vi "Safety_Check.vi"(1 "Adam Loop Count":i32, 2 "Ch Names":string[](array[string]), 3 "Values":dbl[](array[numeric]) format="%.2f") -> (0 "Scan comment":string)   [LabVIEW 2012]
uses:
  ADAM Client/Sub VIs/ADAM Controls/Update_scan_value.ctl
  Anemometry/Anemometry Sub Vis/Globals/Gas_management_global.vi
  ADAM_Global.vi
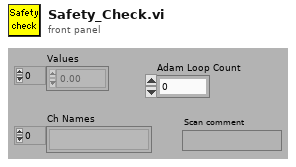
[diagram p1: front panel]
types:
  T1 = cluster{"Channel name":string, "Set value of A to":dbl, "Set value of B to":dbl, "Set value of C to":dbl, "Set value of D to":dbl}
  T2 = typedef "Update_scan_value.ctl" = cluster{"Channel Name":string, "New Value":dbl}
  T3 = enum16{"Append to Global", "Read Global then Clear"}
  T4 = enum16{"On", "Off", "Always On", "Always Off", "Delete"}
  T5 = typedef "LVDateTimeRec.ctl" = cluster{"fractional second":dbl, "second":i32, "minute":i32, "hour":i32, "day of month":i32, "month":i32, "year":i32, "day of week":i32, "day of year":i32, "DST":i32}
  T6 = cluster{"Channel name":string, "Set value of A to":dbl, "Set value of B to":dbl, "Set value of C to":dbl, "Set value of D to":dbl}[]
  T7 = typedef "Ch_description_ADAM.ctl" = cluster{"Ch Name":string, "Type":T8, "Function":T9, "Ch State":T10, "Calibration type":T11, "A":dbl, "B":dbl, "C":dbl, "D":dbl, "Comments":string, "Address":T12, "String":string, "Duty":u16}
  T8 = typedef "Module_type_ADAM.ctl" = string
  T9 = typedef "Function_ADAM.ctl" = enum16{"Analogue Input", "Digital Input", "Event counter", "Event rate", "Analogue Output", "Digital Output", "Relay Output"}
  T10 = typedef "Channel_State.ctl" = enum16{"On", "Off", "Always On", "Always Off"}
  T11 = typedef "Calib_type_ADAM.ctl" = enum16{"Raw", "Bx + A", "Cx^2 + Bx + A", "Dx^3 + Cx^2 + Bx + A", "In Band", "Hi-Tec Q", "Hi-Tec M_dot", "Text"}
  T12 = typedef "Address.ctl" = cluster{"Main":i32, "Ch.":i32, "Sub":i32, "Port Name":string}
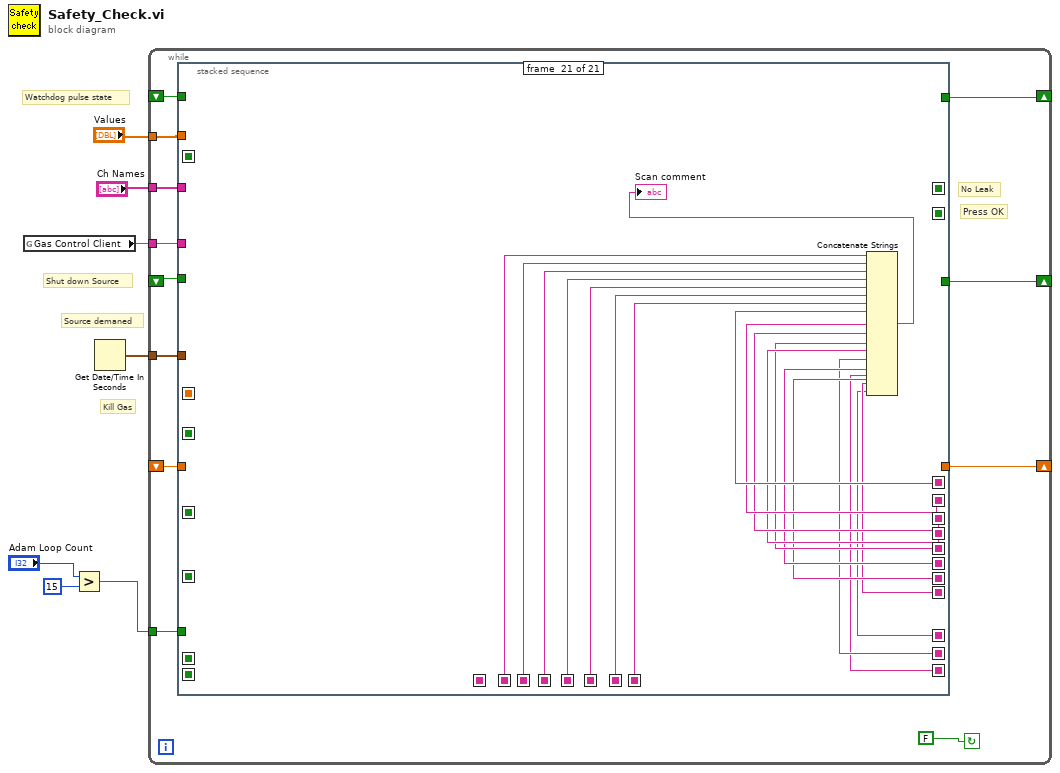
[diagram p0: block diagram]
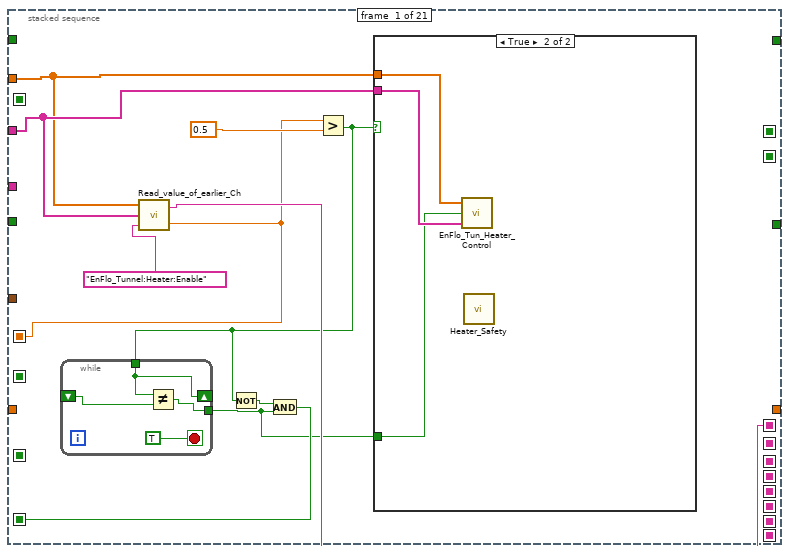
[diagram p2: hidden frame]
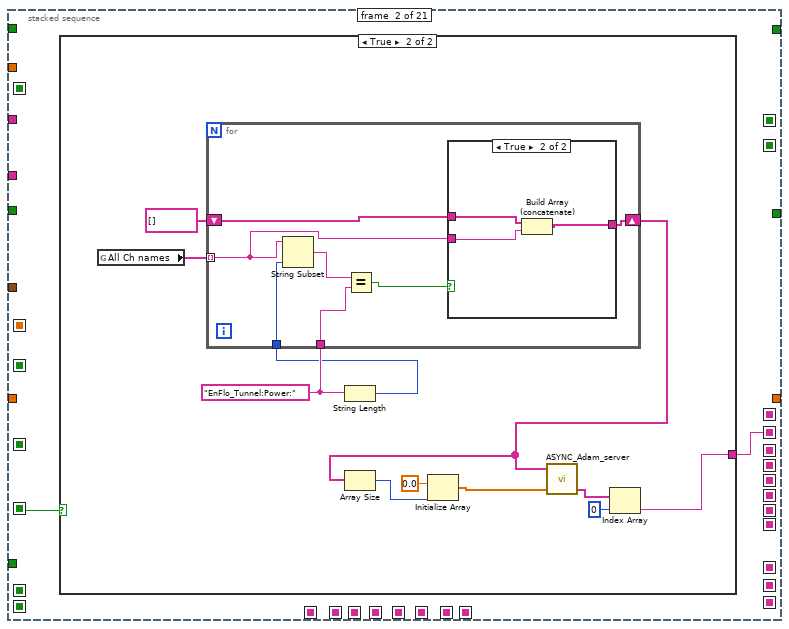
[diagram p4: hidden frame]
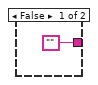
[diagram p5: hidden frame]
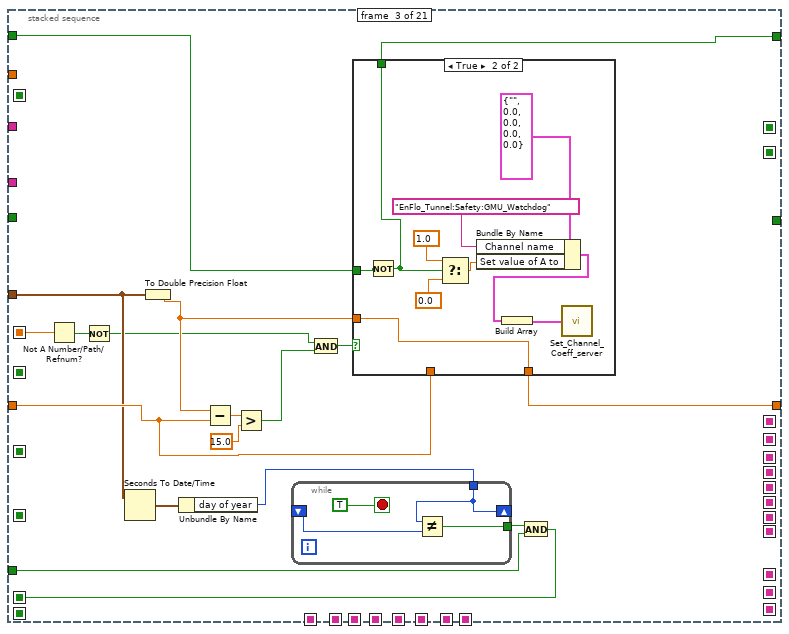
[diagram p7: hidden frame]
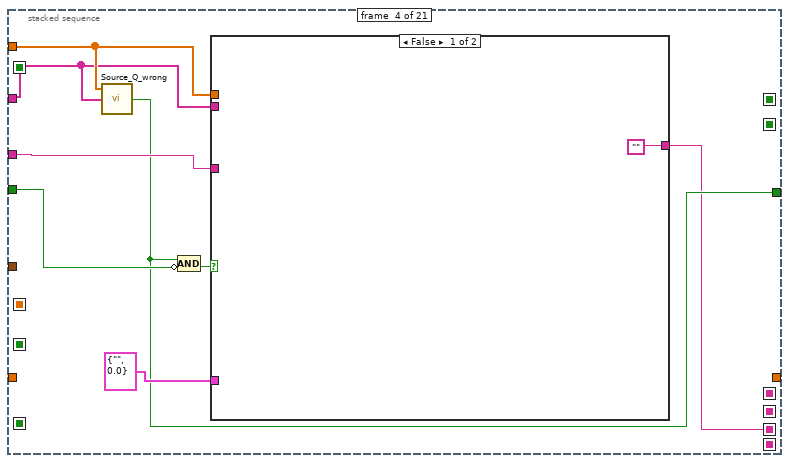
[diagram p9: hidden frame]
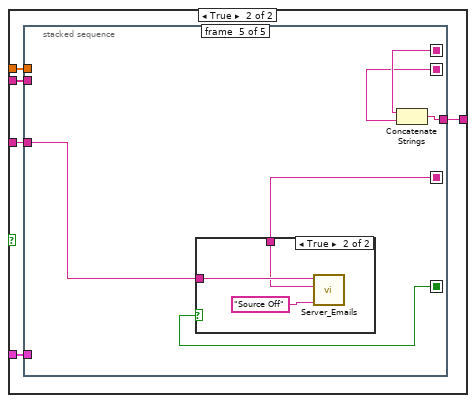
[diagram p10: hidden frame]
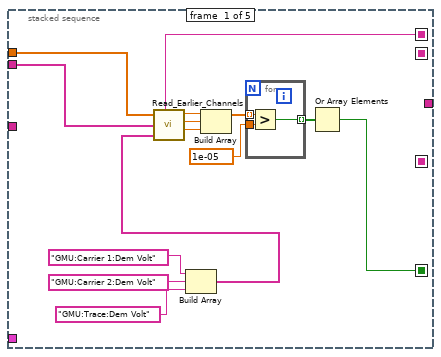
[diagram p11: hidden frame]
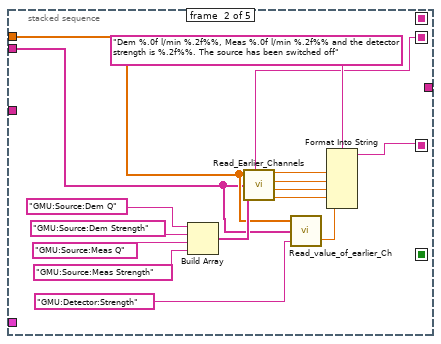
[diagram p12: hidden frame]
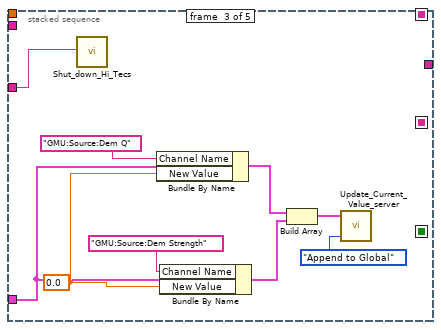
[diagram p13: hidden frame]
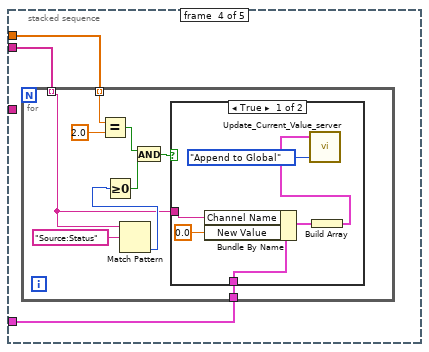
[diagram p14: hidden frame]
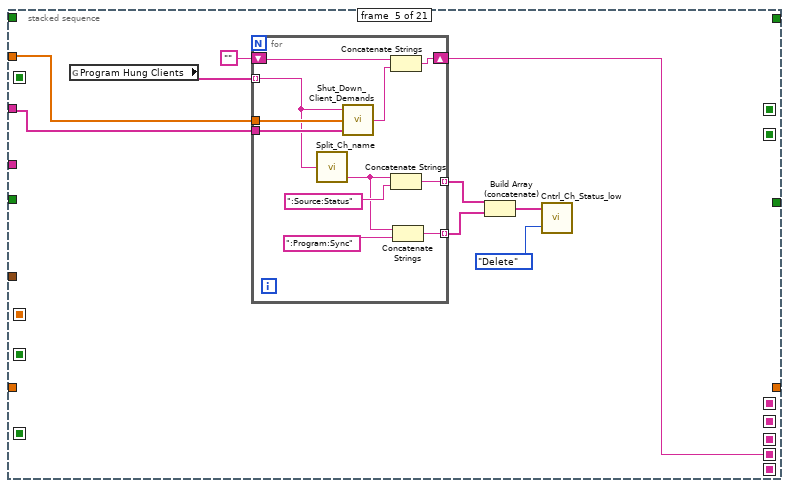
[diagram p17: hidden frame]
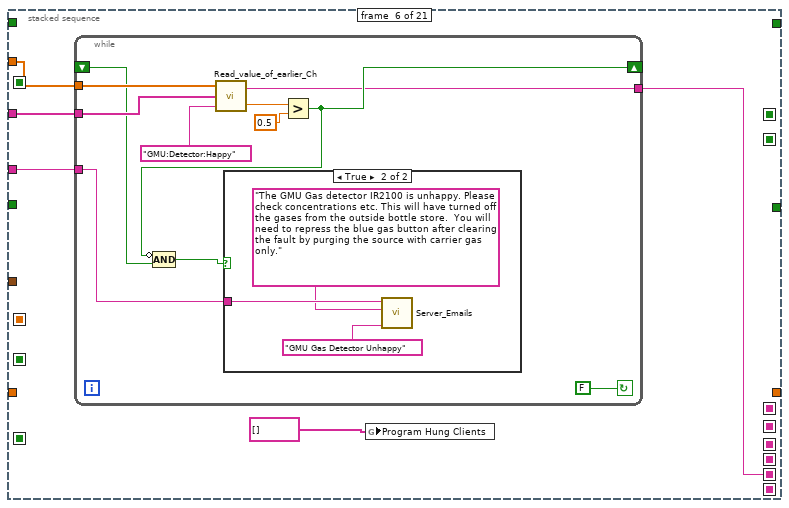
[diagram p18: hidden frame]
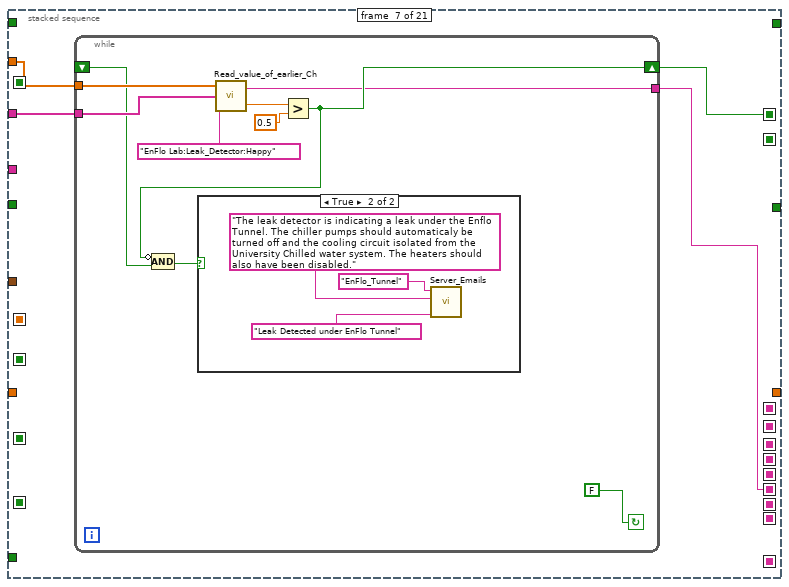
[diagram p20: hidden frame]
diagram:
  # "Shut down Source"
  # "Source demaned"
  # "Watchdog pulse state"
  # "Kill Gas"
  n1 = global read "Gas_management_global.vi" "Gas Control Client"() -> (w5:string)
  n2 = Greater?(x="Adam Loop Count", y=15) -> (0:w2:bool)
  n3 = Get Date/Time In Seconds() -> (seconds since 1Jan1904=w1:timestamp)
  n4 = while {
    shift-left: _ -> [w14]
    shift-right: [w13] -> _
    shift-left: _ -> [w16]
    shift-right: [w15] -> _
    tunnel: w5 -> [w18]
    tunnel: "Ch Names" -> [w19]
    tunnel: "Values" -> [w17]
    shift-right: [w11] -> _
    shift-left: _ -> [w10]
    tunnel: w2 -> [w9]
    tunnel: w1 -> [w8]
    stop <- FALSE continue-if-true
    # "Press OK"
    # "No Leak"
    n5 = stacked-sequence {
      seq-local: [_ _ _ _ _ _ w219 _ _ _ _ _ _ _ _ _ _ _ _ _ _] -> [_ _ _ _ _ _ _ _ _ _ _ _ _ w448 _ _ _ _ _ _ _]
      seq-local: [w22 _ _ _ _ _ _ _ _ _ _ _ _ _ _ _ _ _ _ _ _] -> [_ w38 _ _ _ _ _ _ _ _ _ _ _ _ _ _ _ _ _ _ _]
      seq-local: [_ _ w68 _ _ _ _ _ _ _ _ _ _ _ _ _ _ _ _ _ _] -> [_ _ _ _ _ _ _ _ _ _ _ _ _ _ _ _ _ _ _ _ _]
      seq-local: [_ _ _ _ _ _ _ _ _ _ _ _ _ _ _ w509 _ _ _ _ _] -> [_ _ _ _ _ _ _ _ _ _ _ _ _ _ _ _ w525 _ _ _ _]
      seq-local: [_ _ _ _ _ _ _ _ _ _ _ _ _ _ _ _ w517 _ _ _ _] -> [_ _ _ _ _ _ _ _ _ _ _ _ _ _ _ _ _ _ _ w649 _]
      seq-local: [w25 _ _ _ _ _ _ _ _ _ _ _ _ _ _ _ _ _ _ _ _] -> [_ _ _ _ _ _ _ _ _ _ _ _ _ _ _ _ _ _ _ _ w686]
      seq-local: [_ w37 _ _ _ _ _ _ _ _ _ _ _ _ _ _ _ _ _ _ _] -> [_ _ _ _ _ _ _ _ _ _ _ _ _ _ _ _ _ _ _ _ w685]
      seq-local: [_ _ _ w96 _ _ _ _ _ _ _ _ _ _ _ _ _ _ _ _ _] -> [_ _ _ _ _ _ _ _ _ _ _ _ _ _ _ _ _ _ _ _ w684]
      seq-local: [_ _ _ _ w179 _ _ _ _ _ _ _ _ _ _ _ _ _ _ _ _] -> [_ _ _ _ _ _ _ _ _ _ _ _ _ _ _ _ _ _ _ _ w683]
      seq-local: [_ _ _ _ _ w199 _ _ _ _ _ _ _ _ _ _ _ _ _ _ _] -> [_ _ _ _ _ _ _ _ _ _ _ _ _ _ _ _ _ _ _ _ w682]
      seq-local: [_ _ _ _ _ _ w218 _ _ _ _ _ _ _ _ _ _ _ _ _ _] -> [_ _ _ _ _ _ _ _ _ _ _ _ _ _ _ _ _ _ _ _ w681]
      seq-local: [_ _ _ _ _ _ _ _ _ w326 _ _ _ _ _ _ _ _ _ _ _] -> [_ _ _ _ _ _ _ _ _ _ _ _ _ _ _ _ _ _ _ _ w680]
      seq-local: [_ _ _ _ _ _ _ _ _ _ w358 _ _ _ _ _ _ _ _ _ _] -> [_ _ _ _ _ _ _ _ _ _ _ _ _ _ _ _ _ _ _ _ w671]
      seq-local: [_ _ _ _ _ _ _ _ _ _ _ _ w425 _ _ _ _ _ _ _ _] -> [_ _ _ _ _ _ _ _ _ _ _ _ _ _ _ _ _ _ _ _ w670]
      seq-local: [_ _ _ _ _ _ _ _ _ _ _ _ _ w449 _ _ _ _ _ _ _] -> [_ _ _ _ _ _ _ _ _ _ _ _ _ _ _ _ _ _ _ _ w673]
      seq-local: [_ _ _ _ _ _ _ _ _ _ _ _ _ _ w476 _ _ _ _ _ _] -> [_ _ _ _ _ _ _ _ _ _ _ _ _ _ _ _ _ _ _ _ w674]
      seq-local: [_ _ _ _ _ _ _ _ _ _ _ _ _ _ _ w500 _ _ _ _ _] -> [_ _ _ _ _ _ _ _ _ _ _ _ _ _ _ _ _ _ _ _ w675]
      seq-local: [_ _ _ _ _ _ _ _ _ _ _ _ _ _ _ _ w514 _ _ _ _] -> [_ _ _ _ _ _ _ _ _ _ _ _ _ _ _ _ _ _ _ _ w676]
      seq-local: [_ _ _ _ _ _ _ _ _ _ _ _ _ _ _ _ _ w582 _ _ _] -> [_ _ _ _ _ _ _ _ _ _ _ _ _ _ _ _ _ _ _ _ w677]
      seq-local: [_ _ _ _ _ _ _ _ _ _ _ _ _ _ _ _ _ _ w611 _ _] -> [_ _ _ _ _ _ _ _ _ _ _ _ _ _ _ _ _ _ _ _ w678]
      seq-local: [_ _ _ _ _ _ _ _ _ _ _ _ _ _ _ _ _ _ _ w647 _] -> [_ _ _ _ _ _ _ _ _ _ _ _ _ _ _ _ _ _ _ _ w679]
      seq-local: [w24 _ _ _ _ _ _ _ _ _ _ _ _ _ _ _ _ _ _ _ _] -> [_ _ w66 _ _ _ _ _ _ _ _ _ _ _ _ _ _ _ _ _ _]
      seq-local: [_ _ _ _ _ _ _ _ _ _ _ _ _ _ _ w499 _ _ _ _ _] -> [_ _ _ _ _ _ _ _ _ _ _ _ _ _ _ _ w513 _ _ _ _]
      seq-local: [_ _ _ _ _ _ _ w237 _ _ _ _ _ _ _ _ _ _ _ _ _] -> [_ _ _ _ _ _ _ _ _ _ _ _ _ w447 _ _ _ _ _ _ _]
      seq-local: [_ _ _ _ _ _ _ w236 _ _ _ _ _ _ _ _ _ _ _ _ _] -> [_ _ _ _ _ _ _ _ _ _ _ _ _ _ _ _ _ _ _ _ w669]
      seq-local: [_ _ _ _ _ _ _ w235 _ _ _ _ _ _ _ _ _ _ _ _ _] -> [_ _ _ _ _ _ _ _ w267 _ _ _ _ _ _ _ _ _ _ _ _]
      seq-local: [_ _ _ _ _ _ _ _ w264 _ _ _ _ _ _ _ _ _ _ _ _] -> [_ _ _ _ _ _ _ _ _ _ _ _ _ _ _ _ _ _ _ _ _]
      seq-local: [_ _ _ _ _ _ _ _ _ _ _ w379 _ _ _ _ _ _ _ _ _] -> [_ _ _ _ _ _ _ _ _ _ _ _ _ _ _ _ _ _ _ _ w668]
      tunnel: w19 -> [w27 _ _ w98 w186 w201 w220 w238 w265 w327 w359 w380 w427 w450 w482 w505 w526 w587 w614 _ _]
      tunnel: w18 -> [_ _ _ w103 _ w200 _ _ _ _ _ _ _ _ _ _ _ _ _ _ _]
      tunnel: w17 -> [w26 _ _ w99 w182 w202 w221 w239 w266 w328 w360 w381 w428 w451 w483 w506 w527 w588 w615 _ _]
      tunnel: w16 -> [_ _ w79 _ _ _ _ _ _ _ _ _ _ _ _ _ _ _ _ _ _]
      tunnel: [_ _ w78 _ _ _ _ _ _ _ _ _ _ _ _ _ _ _ _ _ _] -> w15
      tunnel: w14 -> [_ _ _ w102 _ _ _ _ _ _ _ _ _ _ _ _ _ _ _ _ _]
      tunnel: [_ _ _ w97 _ _ _ _ _ _ _ _ _ _ _ _ _ _ _ _ _] -> w13
      tunnel: [_ _ w77 _ _ _ _ _ _ _ _ _ _ _ _ _ _ _ _ _ _] -> w11
      tunnel: w10 -> [_ _ w73 _ _ _ _ _ _ _ _ _ _ _ _ _ _ _ _ _ _]
      tunnel: w9 -> [_ _ w69 _ _ _ _ _ _ _ _ _ w426 _ _ _ w518 w583 _ w648 _]
      tunnel: w8 -> [_ _ w67 _ _ _ _ _ _ _ _ w378 _ _ _ _ _ _ _ _ _]
      frame #0 {
        n6 = call "Read_value_of_earlier_Ch.vi"("Desired Ch to Read"="EnFlo_Tunnel:Heater:Enable", "Ch names"=w27, "Present scan array"=w26) -> ("Value"=w24:dbl, "Scan comment"=w25:string)  [unwired: 1 in]
        n7 = Greater?(x=w24, y=0.5) -> (0:w23:bool)
        n8 = while {
          shift-right: [w33] -> _
          shift-left: _ -> [w32]
          tunnel: w23 -> [w33]
          tunnel: [w30] -> w20
          stop <- TRUE stop-if-true
          n9 = Not Equal?(x=w33, y=w32) -> (x != y?=w30:bool)
        }
        n10 = Not(x=w23) -> (.not. x?=w21:bool)
        n11 = And(x=w21, y=w20) -> (x .and. y?=w22:bool)
        n12 = case shown="True" w23 {
          tunnel: w26 -> [_ w36]
          tunnel: w27 -> [_ w35]
          tunnel: w20 -> [_ w34]
          frame False {
          }
          frame True {
            n13 = call "EnFlo_Tun_Heater_Control.vi"("Ch Names"=w35, "Heaters Just Enabled"=w34, "Values"=w36) -> ()  [unwired: 1 in]
            n14 = call "Heater_Safety.vi"() -> ()  [unwired: 3 in, 5 out]
          }
        }
      }
      frame #1 {
        n15 = case shown="True" w38 {
          tunnel: ["" w41] -> w37
          frame False {
          }
          frame True {
            w50 = "EnFlo_Tunnel:Power:"
            n16 = global read "ADAM_Global.vi" "All Ch names"() -> (w40:string[])
            n17 = String Length(string=w50) -> (length=w49:i32)
            n18 = for {
              shift-right: [w52] -> w45
              shift-left: string[] [] -> [w53]
              tunnel: w40 -> [w56] mode=indexing
              tunnel: w49 -> [w57]
              tunnel: w50 -> [w54]
              n19 = String Subset(string=w56, length (rest)=w57) -> (substring=w55:string)  [unwired: 1 out]
              n20 = Equal?(x=w55, y=w54) -> (x = y?=w51:bool)
              n21 = case shown="True" w51 {
                tunnel: w56 -> [_ w61]
                tunnel: w53 -> [w58 w59]
                tunnel: [w58 w60] -> w52
                frame False {
                }
                frame True {
                  n22 = Build Array (concatenate)(w59, w61) -> (w60:string[])
                }
              }
            }
            n23 = Array Size(array=w45) -> (size(s)=w46:i32)
            n24 = Initialize Array(0.0 ("element"), w46) -> (w44:dbl[])
            n25 = call "ASYNC_Adam_server.vi"("Values"=w44, "Channel Names"=w45) -> ("Scan Comments"=w43:string[])  [unwired: 1 in, 2 out]
            n26 = Index Array(array=w43, index=0) -> (element=w41:string)
          }
        }
      }
      frame #2 {
        n27 = Not A Number/Path/Refnum?(number/path/refnum=w66) -> (NaN/Path/Refnum?=w65:bool)
        n28 = Not(x=w65) -> (.not. x?=w63:bool)
        n29 = Seconds To Date/Time(time stamp (now)=w67) -> (date time rec=w72:T5)  [unwired: 1 in]
        n30 = To Double Precision Float(number=w67) -> (double precision float=w76:dbl)
        n31 = Unbundle By Name(w72) -> ("day of year"=w71:i32)
        n32 = Subtract(x=w76, y=w73) -> (x-y=w75:dbl)
        n33 = Greater?(x=w75, y=15.0) -> (0:w64:bool)
        n34 = while {
          shift-right: [w83] -> _
          shift-left: _ -> [w82]
          tunnel: w71 -> [w83]
          tunnel: [w81] -> w70
          stop <- TRUE stop-if-true
          n35 = Not Equal?(x=w83, y=w82) -> (x != y?=w81:bool)
        }
        n36 = And(x=w63, y=w64) -> (x .and. y?=w62:bool)
        n37 = case shown="True" w62 {
          tunnel: w79 -> [w84 w88]
          tunnel: [w84 w87] -> w78
          tunnel: [w85 w86] -> w77
          tunnel: w76 -> [_ w86]
          tunnel: w73 -> [w85 _]
          frame False {
          }
          frame True {
            n38 = Not(x=w88) -> (.not. x?=w87:bool)
            n39 = Select(t=1.0 ("Suction"), s=w87, f=0.0 ("Suction")) -> (s? t:f=w91:dbl)
            n40 = Bundle By Name(cluster=T1 {"Channel name"="", "Set value of A to"=0.0, "Set value of B to"=0.0, "Set value of C to"=0.0, "Set value of D to"=0.0}, "Channel name"="EnFlo_Tunnel:Safety:GMU_Watchdog" ("Desired Ch to Read"), "Set value of A to"=w91) -> (w95:T1)
            n41 = Build Array(w95) -> (w90:T6)
            n42 = call "Set_Channel_Coeff_server.vi"("Set Array"=w90) -> ()
          }
        }
        n43 = And(x=w70, y=w69) -> (x .and. y?=w68:bool)
      }
      frame #3 {
        n44 = call "Source_Q_wrong.vi"("Ch Names"=w98, "Values"=w99) -> ("Gas Error?"=w97:bool)  [unwired: 1 out]
        n45 = Compound Arithmetic op=AND(w97, invert w102) -> (w101:bool)
        n46 = case shown="False" w101 {
          tunnel: w103 -> [_ w109]
          tunnel: w99 -> [_ w108]
          tunnel: w98 -> [_ w107]
          tunnel: T2 {"Channel Name"="", "New Value"=0.0} ("Update Scan Value Cluster") -> [_ w106]
          tunnel: ["" w105] -> w96
          frame False {
          }
          frame True {
            n47 = stacked-sequence {
              seq-local: [_ w141 _ _ _] -> [_ _ _ _ w174]
              seq-local: [w111 _ _ _ _] -> [_ _ _ _ w173]
              seq-local: [w110 _ _ _ _] -> [_ _ _ _ w172]
              seq-local: [_ w127 _ _ _] -> [_ _ _ _ w171]
              tunnel: w109 -> [_ _ w144 _ w175]
              tunnel: w108 -> [w121 w131 _ w153 _]
              tunnel: w107 -> [w122 w130 _ w154 _]
              tunnel: w106 -> [_ _ w143 w152 _]
              tunnel: [_ _ _ _ w170] -> w105
              frame #0 {
                n48 = Build Array("GMU:Carrier 1:Dem Volt", "GMU:Carrier 2:Dem Volt", "GMU:Trace:Dem Volt") -> (w123:string[])
                n49 = call "Read_Earlier_Channels.vi"("Present scan array"=w121, "Ch names"=w122, "Desired Channels"=w123) -> ("Scan comments"=w110:string, "Index 0"=w117:dbl, "Index 1"=w116:dbl, "Index 2"=w115:dbl)  [unwired: 2 out]
                n50 = Build Array(w117, w116, w115) -> (w114:dbl[])
                n51 = for {
                  tunnel: w114 -> [w126] mode=indexing
                  tunnel: 1e-05 -> [w125]
                  tunnel: [w124] -> w112 mode=indexing
                  n52 = Greater?(x=w126, y=w125) -> (0:w124:bool)
                }
                n53 = Or Array Elements(Boolean array=w112) -> (logical OR=w111:bool)
              }
              frame #1 {
                n54 = Build Array("GMU:Source:Dem Q", "GMU:Source:Dem Strength", "GMU:Source:Meas Q", "GMU:Source:Meas Strength") -> (w136:string[])
                n55 = call "Read_Earlier_Channels.vi"("Present scan array"=w131, "Ch names"=w130, "Desired Channels"=w136) -> ("Scan comments"=w127:string, "Index 0"=w135:dbl, "Index 1"=w134:dbl, "Index 2"=w133:dbl, "Index 3"=w132:dbl)  [unwired: 1 out]
                n56 = call "Read_value_of_earlier_Ch.vi"("Desired Ch to Read"="GMU:Detector:Strength", "Ch names"=w130, "Present scan array"=w131) -> ("Value"=w128:dbl)  [unwired: 1 in, 1 out]
                n57 = Format Into String(format string="Dem %.0f l/min %.2f%%, Meas %.0f l/min %.2f%% and the detector strength is %.2f%%. The source has been switched off" ("Format String"), w135, w134, w133, w132, w128) -> (resulting string=w141:string)  [unwired: 2 in, 1 out]
              }
              frame #2 {
                w145 = 0.0 ("Bundle Element")
                n58 = call "Shut_down_Hi_Tecs.vi"("Client Name"=w144) -> ()  [unwired: 6 out]
                n59 = Bundle By Name(cluster=w143, "Channel Name"="GMU:Source:Dem Q", "New Value"=w145) -> (w150:T2)
                n60 = Bundle By Name(cluster=w143, "Channel Name"="GMU:Source:Dem Strength", "New Value"=w145) -> (w151:T2)
                n61 = Build Array(w150, w151) -> (w147:T2[])
                n62 = call "Update_Current_Value_server.vi"("Mode"=T3."Append to Global", "Update array in"=w147) -> ()  [unwired: 1 in, 1 out]
              }
              frame #3 {
                n63 = for {
                  tunnel: w154 -> [w155] mode=indexing
                  tunnel: w153 -> [w161] mode=indexing
                  tunnel: w152 -> [w156]
                  n64 = Equal?(x=w161, y=2.0) -> (x = y?=w158:bool)
                  n65 = Match Pattern(string=w155, regular expression="Source:Status") -> (offset past match=w162:i32)  [unwired: 4 out]
                  n66 = Greater Or Equal To 0?(x=w162) -> (x >= 0?=w159:bool)
                  n67 = And(x=w158, y=w159) -> (x .and. y?=w157:bool)
                  n68 = case shown="True" w157 {
                    tunnel: w156 -> [w169 _]
                    tunnel: w155 -> [w168 _]
                    frame True {
                      n69 = Bundle By Name(cluster=w169, "Channel Name"=w168, "New Value"=0.0) -> (w166:T2)
                      n70 = Build Array(w166) -> (w165:T2[])
                      n71 = call "Update_Current_Value_server.vi"("Mode"=T3."Append to Global", "Update array in"=w165) -> ()  [unwired: 1 in, 1 out]
                    }
                    frame False {
                    }
                  }
                }
              }
              frame #4 {
                n72 = case shown="True" w173 {
                  tunnel: w175 -> [_ w178]
                  tunnel: w174 -> [_ w177]
                  frame False {
                  }
                  frame True {
                    n73 = call "Server_Emails.vi"("Client Name Contains"=w178, "Message"=w177, "Subject"="Source Off") -> ()  [unwired: 2 in, 3 out]
                  }
                }
                n74 = Concatenate Strings(w172, w171) -> (w170:string)
              }
            }
          }
        }
      }
      frame #4 {
        n75 = global read "ADAM_Global.vi" "Program Hung Clients"() -> (w187:string[])
        n76 = for {
          tunnel: w187 -> [w196] mode=indexing
          tunnel: w182 -> [w198]
          tunnel: w186 -> [w197]
          tunnel: [w194] -> w185 mode=indexing
          tunnel: [w191] -> w184 mode=indexing
          shift-right: [w189] -> w179
          shift-left: "" -> [w190]
          n77 = call "Split_Ch_name.vi"("Ch name"=w196) -> ("Low level"=w193:string)  [unwired: 2 out]
          n78 = call "Shut_Down_Client_Demands.vi"("Ch Names"=w197, "Values"=w198, "Client Name"=w196) -> ("Comments"=w188:string)
          n79 = Concatenate Strings(w190, w188) -> (w189:string)
          n80 = Concatenate Strings(w193, ":Source:Status") -> (w194:string)
          n81 = Concatenate Strings(w193, ":Program:Sync") -> (w191:string)
        }
        n82 = Build Array (concatenate)(w185, w184) -> (w183:string[])
        n83 = call "Cntrl_Ch_Status_low.vi"("Mode"=T4."Delete", "Channel names"=w183) -> ()  [unwired: 1 out]
      }
      frame #5 {
        n84 = while {
          tunnel: w202 -> [w214]
          tunnel: w201 -> [w213]
          shift-right: [w208] -> _
          shift-left: _ -> [w209]
          tunnel: w200 -> [w206]
          tunnel: [w204] -> w199
          stop <- FALSE continue-if-true
          n85 = call "Read_value_of_earlier_Ch.vi"("Desired Ch to Read"="GMU:Detector:Happy", "Ch names"=w213, "Present scan array"=w214) -> ("Value"=w211:dbl, "Scan comment"=w204:string)  [unwired: 1 in]
          n86 = Greater?(x=w211, y=0.5) -> (0:w208:bool)
          n87 = Compound Arithmetic op=AND(invert w208, w209) -> (w207:bool)
          n88 = case shown="True" w207 {
            tunnel: w206 -> [_ w216]
            frame False {
            }
            frame True {
              n89 = call "Server_Emails.vi"("Client Name Contains"=w216, "Message"="The GMU Gas detector IR2100 is unhappy. Please check concentrations etc. This will have turned off the gases from the outside bottle store.  You will need to repress the blue gas button after clearing the fault by purging the source with carrier gas only.", "Subject"="GMU Gas Detector Unhappy") -> ()  [unwired: 2 in, 3 out]
            }
          }
        }
        n90 = global write "ADAM_Global.vi" "Program Hung Clients"(string[] [] ("Program Hung Clients")) -> ()
      }
      frame #6 {
        n91 = while {
          tunnel: w221 -> [w231]
          tunnel: w220 -> [w230]
          shift-right: [w225] -> w219
          shift-left: _ -> [w226]
          tunnel: [w222] -> w218
          stop <- FALSE continue-if-true
          n92 = call "Read_value_of_earlier_Ch.vi"("Desired Ch to Read"="EnFlo Lab:Leak_Detector:Happy", "Ch names"=w230, "Present scan array"=w231) -> ("Value"=w228:dbl, "Scan comment"=w222:string)  [unwired: 1 in]
          n93 = Greater?(x=w228, y=0.5) -> (0:w225:bool)
          n94 = Compound Arithmetic op=AND(invert w225, w226) -> (w224:bool)
          n95 = case shown="True" w224 {
            frame False {
            }
            frame True {
              n96 = call "Server_Emails.vi"("Client Name Contains"="EnFlo_Tunnel", "Message"="The leak detector is indicating a leak under the Enflo Tunnel. The chiller pumps should automaticaly be turned off and the cooling circuit isolated from the  University Chilled water system. The heaters should also have been disabled.", "Subject"="Leak Detected under EnFlo Tunnel") -> ()  [unwired: 2 in, 3 out]
            }
          }
        }
      }
      frame #7 {
        n97 = while {
          tunnel: w239 -> [w245]
          tunnel: w238 -> [w244]
          shift-right: [w256] -> w237
          shift-left: _ -> [w257]
          tunnel: [w248] -> w236
          tunnel: [w240] -> w235
          stop <- FALSE continue-if-true
          n98 = call "Read_value_of_earlier_Ch.vi"("Desired Ch to Read"="EnFlo_Tunnel:Chiller_Pump:Enable", "Ch names"=w244, "Present scan array"=w245) -> ("Value"=w251:dbl, "Scan comment"=w249:string)  [unwired: 1 in]
          n99 = call "Read_value_of_earlier_Ch.vi"("Desired Ch to Read"="EnFlo_Tunnel:Chilled Water:Pressure_OK", "Ch names"=w244, "Present scan array"=w245) -> ("Value"=w259:dbl, "Scan comment"=w250:string)  [unwired: 1 in]
          n100 = call "Read_value_of_earlier_Ch.vi"("Desired Ch to Read"="EnFlo_Tunnel:Chiller_Pump:Running", "Ch names"=w244, "Present scan array"=w245) -> ("Value"=w242:dbl, "Scan comment"=w241:string)  [unwired: 1 in]
          n101 = Greater?(x=w259, y=0.5) -> (0:w256:bool)
          n102 = Greater?(x=w251, y=0.5) -> (0:w247:bool)
          n103 = Compound Arithmetic op=AND(invert w256, w257, w247) -> (w255:bool)
          n104 = case shown="True" w255 {
            frame False {
            }
            frame True {
              n105 = call "Server_Emails.vi"("Client Name Contains"="EnFlo_Tunnel", "Message"="The pressure in the chilled water  for the Enflo Tunnel has tripped the system. The chiller pumps should automaticaly be turned off and the cooling circuit isolated from the  University Chilled water system. The heaters should also have been disabled.", "Subject"="EnFlo Chilled Water Overpressure Trip") -> ()  [unwired: 2 in, 3 out]
            }
          }
          n106 = Greater?(x=w242, y=0.5) -> (0:w240:bool)
          n107 = Concatenate Strings(w249, w250, w241) -> (w248:string)
        }
      }
      frame #8 {
        n108 = case shown="True" w267 {
          tunnel: w266 -> [_ w296]
          tunnel: w265 -> [_ w295]
          tunnel: ["" w269] -> w264
          frame False {
          }
          frame True {
            w274 = "EnFlo_Tunnel:Chilled Water:Motor_Dem_Voltage"
            # "EnFlo_Tunnel:Chiller_Pump:Running"
            n109 = call "Read_value_of_earlier_Ch.vi"("Desired Ch to Read"="EnFlo_Tunnel:Chilled Water:Pressure_supply (Bar)", "Ch names"=w295, "Present scan array"=w296) -> ("Value"=w281:dbl, "Scan comment"=w273:string)  [unwired: 1 in]
            n110 = call "Read_value_of_earlier_Ch.vi"("Desired Ch to Read"="EnFlo_Tunnel:Chilled Water:Pressure_return (Bar)", "Ch names"=w295, "Present scan array"=w296) -> ("Value"=w291:dbl, "Scan comment"=w272:string)  [unwired: 1 in]
            n111 = call "Read_value_of_earlier_Ch.vi"("Desired Ch to Read"="EnFlo_Tunnel:Chilled Water:Desired_Delta_P", "Ch names"=w295, "Present scan array"=w296) -> ("Value"=w289:dbl, "Scan comment"=w271:string)  [unwired: 1 in]
            n112 = call "Read_value_of_earlier_Ch.vi"("Desired Ch to Read"=w274, "Ch names"=w295, "Present scan array"=w296) -> ("Value"=w279:dbl, "Scan comment"=w270:string)  [unwired: 1 in]
            n113 = Subtract(x=w281, y=w291) -> (x-y=w290:dbl)
            n114 = Subtract(x=w290, y=w289) -> (x-y=w277:dbl)
            n115 = Concatenate Strings(w273, w272, w271, w270) -> (w269:string)
            n116 = In Range and Coerce(upper limit=0.1 ("lower limit"), x=w277, lower limit=-0.1) -> (In Range?=w284:bool)  [unwired: 1 out]
            n117 = Less?(x=w281, y=3.9) -> (x < y?=w285:bool)
            n118 = Select(t=w284, s=w285, f=TRUE) -> (s? t:f=w278:bool)
            n119 = Less?(x=w281, y=4.0) -> (x < y?=w280:bool)
            n120 = case shown="True" w280 {
              tunnel: w279 -> [w307 w310]
              tunnel: w278 -> [_ w312]
              tunnel: w277 -> [_ w311]
              tunnel: [TRUE w309] -> w276
              tunnel: [w304 w308] -> w275
              frame False {
                n121 = Subtract(x=w307, y=0.2) -> (x-y=w304:dbl)
              }
              frame True {
                n122 = case shown="False" w312 {
                  tunnel: w311 -> [w317 _]
                  tunnel: w310 -> [w316 w324]
                  tunnel: [TRUE FALSE] -> w309
                  tunnel: [w314 w324] -> w308
                  frame False {
                    n123 = Greater Than 0?(x=w317) -> (x > 0?=w315:bool)
                    n124 = case shown="False" w315 {
                      tunnel: w316 -> [w319 w322]
                      tunnel: [w318 w321] -> w314
                      frame True {
                        n125 = Subtract(x=w319, y=0.1) -> (x-y=w318:dbl)
                      }
                      frame False {
                        n126 = Add(x=w322, y=0.1) -> (x+y=w321:dbl)
                      }
                    }
                  }
                  frame True {
                  }
                }
              }
            }
            n127 = case shown="True" w276 {
              tunnel: w275 -> [_ w298]
              tunnel: w274 -> [_ w301]
              frame False {
              }
              frame True {
                n128 = In Range and Coerce(upper limit=10.0, x=w298, lower limit=0.0) -> (coerced(x)=w297:dbl)  [unwired: 1 out]
                n129 = Build Array(w301) -> (w302:string[])
                n130 = Build Array(w297) -> (w303:dbl[])
                n131 = call "ASYNC_Adam_server.vi"("Values"=w303, "Channel Names"=w302) -> ()  [unwired: 1 in, 3 out]
              }
            }
          }
        }
      }
      frame #9 {
        n132 = while {
          tunnel: w328 -> [w344]
          tunnel: w327 -> [w343]
          shift-right: [w337] -> _
          shift-left: _ -> [w333]
          tunnel: [w329] -> w326
          stop <- FALSE continue-if-true
          w335 = 60.0 ("y")
          n133 = Decrement(x=w335) -> (x-1=w336:dbl)
          n134 = Select(t=w336, s=w333, f=w335) -> (s? t:f=w334:dbl)
          n135 = call "Read_value_of_earlier_Ch.vi"("Desired Ch to Read"="EnFlo_Tunnel:Chilled Water:Motor1 Temp", "Ch names"=w343, "Present scan array"=w344) -> ("Value"=w351:dbl, "Scan comment"=w331:string)  [unwired: 1 in]
          n136 = call "Read_value_of_earlier_Ch.vi"("Desired Ch to Read"="EnFlo_Tunnel:Chilled Water:Motor2 Temp", "Ch names"=w343, "Present scan array"=w344) -> ("Value"=w348:dbl, "Scan comment"=w330:string)  [unwired: 1 in]
          n137 = Greater?(x=w351, y=w334) -> (0:w345:bool)
          n138 = Greater?(x=w348, y=w334) -> (0:w346:bool)
          n139 = Or(x=w345, y=w346) -> (x .or. y?=w339:bool)
          n140 = call "Read_value_of_earlier_Ch.vi"("Desired Ch to Read"="EnFlo_Tunnel:Chiller_Pump:Enable", "Ch names"=w343, "Present scan array"=w344) -> ("Value"=w341:dbl, "Scan comment"=w332:string)  [unwired: 1 in]
          n141 = Greater?(x=w341, y=0.5) -> (0:w338:bool)
          n142 = And(x=w338, y=w339) -> (x .and. y?=w337:bool)
          n143 = Compound Arithmetic op=AND(w337, invert w333) -> (w350:bool)
          n144 = case shown="True" w350 {
            tunnel: w335 -> [_ w354]
            frame False {
            }
            frame True {
              n145 = Format Into String(format string="The Chilled Water Motor Temp is greater than %.0f deg C." ("Message"), w354) -> (resulting string=w353:string)  [unwired: 2 in, 1 out]
              n146 = call "Server_Emails.vi"("Client Name Contains"="EnFlo_Tunnel", "Message"=w353, "Subject"="Chilled Water Motor Temp") -> ()  [unwired: 2 in, 3 out]
            }
          }
          n147 = Concatenate Strings(w332, w331, w330) -> (w329:string)
        }
      }
      frame #10 {
        n148 = while {
          tunnel: w360 -> [w374]
          tunnel: w359 -> [w373]
          shift-right: [w362] -> _
          shift-left: _ -> [w368]
          shift-left: _ -> [w367]
          shift-left: _ -> [w366]
          tunnel: [w361] -> w358
          stop <- FALSE continue-if-true
          n149 = call "Read_value_of_earlier_Ch.vi"("Desired Ch to Read"="FFID:System:Enable", "Ch names"=w373, "Present scan array"=w374) -> ("Value"=w369:dbl, "Scan comment"=w361:string)  [unwired: 1 in]
          n150 = Greater?(x=w369, y=0.5) -> (0:w362:bool)
          n151 = Compound Arithmetic op=AND(w362, w368, invert w367, invert w366) -> (w364:bool)
          n152 = Compound Arithmetic op=AND(invert w362, invert w368, w367, w366) -> (w365:bool)
          n153 = Or(x=w364, y=w365) -> (x .or. y?=w363:bool)
          n154 = case shown="False" w363 {
            tunnel: w369 -> [_ w375]
            tunnel: w362 -> [_ _]
            frame False {
            }
            frame True {
              n155 = Build Array(w375) -> (w377:dbl[])
              n156 = call "ASYNC_Adam_server.vi"("Values"=w377, "Channel Names"=string[] ["GMU:Gas:Enable"]) -> ()  [unwired: 1 in, 3 out]
            }
          }
        }
      }
      frame #11 {
        n157 = while {
          tunnel: w381 -> [w393]
          tunnel: w380 -> [w392]
          shift-right: [w382] -> _
          shift-left: _ -> [w388]
          shift-left: _ -> [w387]
          tunnel: [w386] -> w379
          tunnel: w378 -> [w384]
          stop <- FALSE continue-if-true
          w383 = "EnFlo_Tunnel:Motor:Enable" ("Desired Ch to Read")
          # "Re Zero EnFlo Tunnel static pressure when turning tunnel on"
          n158 = call "Read_value_of_earlier_Ch.vi"("Desired Ch to Read"=w383, "Ch names"=w392, "Present scan array"=w393) -> ("Value"=w389:dbl, "Scan comment"=w386:string)  [unwired: 1 in]
          n159 = Greater?(x=w389, y=0.5) -> (0:w382:bool)
          n160 = Compound Arithmetic op=AND(w382, invert w388, invert w387) -> (w385:bool)
          n161 = case shown="True" w385 {
            tunnel: w384 -> [_ w419]
            tunnel: w383 -> [_ w417]
            frame False {
            }
            frame True {
              w416 = "EnFlo_Tunnel:Pressure:Static"
              n162 = To Double Precision Float(number=w419) -> (double precision float=w402:dbl)
              n163 = Build Array(w416) -> (w415:string[])
              n164 = Build Array(w417, w416) -> (w420:string[])
              n165 = Subtract(x=w402, y=15.0) -> (x-y=w400:dbl)
              n166 = call "Get_Current_Scan_server.vi"("Desired Channels"=w415) -> ("Ch Description Array"=w414:T7[])  [unwired: 2 out]
              n167 = Subtract(x=w402, y=3600.0) -> (x-y=w418:dbl)
              n168 = call "Get_ADAM_averages_server.vi"("No of averages"=600, "End time"=w400, "Start time"=w418, "Clients time"=w402, "ADAM Ch Names"=w420) -> ("DBL values"=w404:dbl[][])  [unwired: 1 in, 4 out]
              n169 = Index Array(array=w414) -> (element=w412:T7)  [unwired: 1 in]
              n170 = Unbundle By Name(w412) -> ("A"=w413:dbl)
              n171 = Index Array(array=w404, index (col)=1 ("disabled index (col)")) -> (element=w399:dbl[])  [unwired: 1 in]
              n172 = Index Array(array=w404, index (col)=2 ("disabled index (col)")) -> (element=w398:dbl[])  [unwired: 1 in]
              n173 = Reverse 1D Array(array=w398) -> (reversed array=w394:dbl[])
              n174 = Reverse 1D Array(array=w399) -> (reversed array=w397:dbl[])
              n175 = for {
                tunnel: w397 -> [w422] mode=indexing
                tunnel: [w421] -> w396 mode=indexing
                tunnel: w394 -> [w421] mode=indexing
                stop <- w423 continue-if-true
                n176 = Less?(x=w422, y=0.01) -> (x < y?=w423:bool)
              }
              n177 = call "Mean_fr_NaN_data.vi"("Data"=w396) -> ("Mean value"=w395:dbl)  [unwired: 1 out]
              n178 = Subtract(x=w413, y=w395) -> (x-y=w411:dbl)
              n179 = Bundle By Name(cluster=w412, "A"=w411) -> (w410:T7)
              n180 = Build Array(w410) -> (w409:T7[])
              n181 = call "Update_Ch_Discription_server.vi"("Mode"=T3."Append to Global", "Channels to update In"=w409) -> ()  [unwired: 1 in, 1 out]
            }
          }
        }
      }
      frame #12 {
        # "Resetting A Tunnel speed to zero if the drive in turned off\nso that the belts do not slip when the tunnel is turned on again."
        n182 = while {
          tunnel: w428 -> [w441]
          tunnel: w427 -> [w440]
          shift-right: [w432] -> _
          shift-left: _ -> [w435]
          shift-left: _ -> [w434]
          shift-left: _ -> [w433]
          tunnel: w426 -> [w431]
          tunnel: [w429] -> w425
          stop <- FALSE continue-if-true
          n183 = call "Read_value_of_earlier_Ch.vi"("Desired Ch to Read"="A_Tunnel:Motor:Enable", "Ch names"=w440, "Present scan array"=w441) -> ("Value"=w436:dbl, "Scan comment"=w429:string)  [unwired: 1 in]
          n184 = Less?(x=w436, y=0.5) -> (x < y?=w432:bool)
          n185 = Compound Arithmetic op=AND(w432, w435, invert w434, invert w433, w431) -> (w430:bool)
          n186 = case shown="True" w430 {
            tunnel: w432 -> [_ _]
            frame False {
            }
            frame True {
              w444 = string[] ["A_Tunnel:Speed:Dem Velocity", "A_Tunnel:Speed:Dem Voltage"] ("Channel Names")
              n187 = Array Size(array=w444) -> (size(s)=w445:i32)
              n188 = Initialize Array(0.0 ("element"), w445) -> (w443:dbl[])
              n189 = call "ASYNC_Adam_server.vi"("Values"=w443, "Channel Names"=w444) -> ()  [unwired: 1 in, 3 out]
            }
          }
        }
      }
      frame #13 {
        n190 = And(x=w447, y=w448) -> (x .and. y?=w446:bool)
        n191 = case shown="False" w446 {
          tunnel: w451 -> [w456 _]
          tunnel: w450 -> [w455 _]
          tunnel: [w452 ""] -> w449
          frame False {
            n192 = for {
              tunnel: w456 -> [w466]
              tunnel: w455 -> [w465]
              tunnel: string[] ["EnFlo_Tunnel:Heater:Enable", "EnFlo_Tunnel:Chiller_Pump:Enable", "EnFlo_Tunnel:Tap_Water:Enable"] ("Ch Names") -> [w461] mode=indexing
              shift-right: [w459] -> w452
              shift-left: "" -> [w460]
              n193 = call "Read_value_of_earlier_Ch.vi"("Desired Ch to Read"=w461, "Ch names"=w465, "Present scan array"=w466) -> ("Value"=w463:dbl, "Scan comment"=w458:string)  [unwired: 1 in]
              n194 = Greater?(x=w463, y=0.5) -> (0:w462:bool)
              n195 = case shown="True" w462 {
                tunnel: w461 -> [_ w471]
                tunnel: ["" w468] -> w457
                frame False {
                }
                frame True {
                  n196 = Build Array(w471) -> (w474:string[])
                  n197 = Build Array(0.0) -> (w473:dbl[])
                  n198 = call "ASYNC_Adam_server.vi"("Values"=w473, "Channel Names"=w474) -> ("Scan Comments"=w469:string[])  [unwired: 1 in, 2 out]
                  n199 = Index Array(array=w469, index=0) -> (element=w468:string)
                }
              }
              n200 = Concatenate Strings(w460, w458, w457) -> (w459:string)
            }
          }
          frame True {
          }
        }
      }
      frame #14 {
        w484 = "EnFlo_Tunnel:Heater:Enable" ("Ch Name")
        n201 = call "Read_value_of_earlier_Ch.vi"("Desired Ch to Read"=w484, "Ch names"=w482, "Present scan array"=w483) -> ("Value"=w489:dbl, "Scan comment"=w478:string)  [unwired: 1 in]
        n202 = call "Read_value_of_earlier_Ch.vi"("Desired Ch to Read"="EnFlo_Tunnel:Reference:Velocity", "Ch names"=w482, "Present scan array"=w483) -> ("Value"=w486:dbl, "Scan comment"=w477:string)  [unwired: 1 in]
        n203 = Greater?(x=w489, y=0.5) -> (0:w481:bool)
        n204 = Less?(x=w486, y=0.25) -> (x < y?=w485:bool)
        n205 = And(x=w481, y=w485) -> (x .and. y?=w480:bool)
        n206 = case shown="True" w480 {
          tunnel: w484 -> [_ w495]
          tunnel: ["" w492] -> w479
          frame False {
          }
          frame True {
            n207 = Build Array(w495) -> (w498:string[])
            n208 = Build Array(0.0) -> (w497:dbl[])
            n209 = call "ASYNC_Adam_server.vi"("Values"=w497, "Channel Names"=w498) -> ("Scan Comments"=w493:string[])  [unwired: 1 in, 2 out]
            n210 = Index Array(array=w493, index=0) -> (element=w492:string)
          }
        }
        n211 = Concatenate Strings(w478, w477, w479) -> (w476:string)
      }
      frame #15 {
        n212 = call "Read_value_of_earlier_Ch.vi"("Desired Ch to Read"="EnFlo_Tunnel:Chiller_Pump:Running", "Ch names"=w505, "Present scan array"=w506) -> ("Value"=w507:dbl, "Scan comment"=w502:string)  [unwired: 1 in]
        n213 = call "Read_value_of_earlier_Ch.vi"("Desired Ch to Read"="EnFlo_Tunnel:Reference:Velocity", "Ch names"=w505, "Present scan array"=w506) -> ("Value"=w503:dbl, "Scan comment"=w501:string)  [unwired: 1 in]
        n214 = Greater?(x=w503, y=0.4) -> (0:w511:bool)
        n215 = Greater?(x=w507, y=0.5) -> (0:w499:bool)
        n216 = Compound Arithmetic op=AND(w499, w511) -> (w509:bool)
        n217 = Concatenate Strings(w502, w501) -> (w500:string)
      }
      frame #16 {
        w523 = "EnFlo_Tunnel:Heat_Ex_Div_Valve:Dem Pos"
        n218 = case shown="True" w525 {
          tunnel: w527 -> [_ w565]
          tunnel: w526 -> [_ w566]
          tunnel: w523 -> [_ w569]
          tunnel: [0.0 ("upper limit") w575] -> w519
          tunnel: ["" w560] -> w516
          frame False {
          }
          frame True {
            n219 = call "Read_value_of_earlier_Ch.vi"("Desired Ch to Read"="EnFlo_Tunnel:Exit Duct:Dem Temp", "Ch names"=w566, "Present scan array"=w565) -> ("Value"=w574:dbl, "Scan comment"=w564:string)  [unwired: 1 in]
            n220 = call "Read_value_of_earlier_Ch.vi"("Desired Ch to Read"="EnFlo_Tunnel:Exit Duct Top:Temp", "Ch names"=w566, "Present scan array"=w565) -> ("Value"=w570:dbl, "Scan comment"=w563:string)  [unwired: 1 in]
            n221 = call "Read_value_of_earlier_Ch.vi"("Desired Ch to Read"="EnFlo_Tunnel:Exit Duct:Temp", "Ch names"=w566, "Present scan array"=w565) -> ("Value"=w571:dbl, "Scan comment"=w562:string)  [unwired: 1 in]
            n222 = call "Read_value_of_earlier_Ch.vi"("Desired Ch to Read"=w569, "Ch names"=w566, "Present scan array"=w565) -> ("Value"=w572:dbl, "Scan comment"=w561:string)  [unwired: 1 in]
            n223 = Add(x=w570, y=w571) -> (x+y=w579:dbl)
            n224 = Divide(x=w579, y=2.0) -> (x/y=w581:dbl)
            n225 = Concatenate Strings(w564, w563, w562, w561) -> (w560:string)
            n226 = call "Back_End_Chiller_PID.vi"("Present Value"=w581, "Previous Control Sum"=w572, "Setpoint"=w574) -> ("Dem Output"=w578:dbl)
            n227 = In Range and Coerce(upper limit=100.0, x=w578, lower limit=0.0) -> (coerced(x)=w575:dbl)  [unwired: 1 out]
          }
        }
        n228 = while {
          shift-right: [w557] -> w524
          shift-left: _ -> [_]
          tunnel: w513 -> [w557]
          shift-left: _ -> [_]
          shift-left: _ -> [_]
          shift-left: _ -> [_]
          shift-left: _ -> [_]
          shift-left: _ -> [_]
          shift-left: _ -> [_]
          shift-left: _ -> [_]
          shift-left: _ -> [_]
          shift-left: _ -> [_]
          shift-left: _ -> [_]
          shift-left: _ -> [_]
          shift-left: _ -> [_]
          shift-left: _ -> [_]
          shift-left: _ -> [_]
          shift-left: _ -> [_]
          shift-left: _ -> [_]
          shift-left: _ -> [w556]
          tunnel: [w556] -> w522
          stop <- TRUE stop-if-true
        }
        n229 = And(x=w524, y=w522) -> (x .and. y?=w521:bool)
        n230 = case shown="False" w521 {
          tunnel: [w529 w540] -> w520
          tunnel: w519 -> [_ w540]
          tunnel: [w528 FALSE] -> w517
          frame False {
            # "Exercise valve once a week"
            n231 = Seconds To Date/Time() -> (date time rec=w530:T5)  [unwired: 2 out]
            n232 = Unbundle By Name(w530) -> ("day of week"=w535:i32, "hour"=w533:i32)
            n233 = Less?(x=w533, y=3) -> (x < y?=w538:bool)
            n234 = Equal?(x=7, y=w535) -> (x = y?=w537:bool)
            n235 = And(x=w537, y=w538) -> (x .and. y?=w528:bool)
            n236 = Select(t=100.0, s=w528, f=0.0) -> (s? t:f=w529:dbl)
          }
          frame True {
          }
        }
        n237 = while {
          shift-right: [w546] -> _
          shift-left: _ -> [w547]
          tunnel: w520 -> [w546]
          tunnel: w523 -> [w548]
          tunnel: w518 -> [w543]
          tunnel: [w541] -> w515
          stop <- TRUE stop-if-true
          n238 = Not Equal?(x=w546, y=w547) -> (x != y?=w544:bool)
          n239 = Compound Arithmetic op=OR(w544, invert w543) -> (w542:bool)
          n240 = Build Array(w548) -> (w549:string[])
          n241 = Build Array(w546) -> (w550:dbl[])
          n242 = case shown="False" w542 {
            tunnel: w550 -> [_ w554]
            tunnel: w549 -> [_ w553]
            tunnel: [string[] [] ("Scan Comments") w552] -> w541
            frame False {
            }
            frame True {
              n243 = call "ASYNC_Adam_server.vi"("Values"=w554, "Channel Names"=w553) -> ("Scan Comments"=w552:string[])  [unwired: 1 in, 2 out]
            }
          }
        }
        n244 = Concatenate Strings(w516, w515) -> (w514:string)
      }
      frame #17 {
        n245 = Search 1D Array(1D array=w587, element="Status:of:EnFlo_Tunnel") -> (index of element=w590:i32)  [unwired: 1 out]
        n246 = Index Array(array=w588, index=w590) -> (element=w586:dbl)
        n247 = case shown="0, Default" w586 {
          tunnel: [0.0 1.0 1.0 1.0] -> w585
          frame 0, Default {
          }
          frame 1 {
          }
          frame 2 {
          }
          frame 3 {
          }
        }
        n248 = while {
          shift-right: [w600] -> _
          shift-left: _ -> [w601]
          tunnel: w585 -> [w600]
          tunnel: "EnFlo_Tunnel:Warning_Cone:Enable" -> [w602]
          tunnel: w583 -> [w597]
          tunnel: [w595] -> w582
          stop <- TRUE stop-if-true
          n249 = Not Equal?(x=w600, y=w601) -> (x != y?=w598:bool)
          n250 = Build Array(w602) -> (w603:string[])
          n251 = Build Array(w600) -> (w604:dbl[])
          n252 = Compound Arithmetic op=OR(w598, invert w597) -> (w596:bool)
          n253 = case shown="True" w596 {
            tunnel: w604 -> [_ w610]
            tunnel: w603 -> [_ w609]
            tunnel: ["" w606] -> w595
            frame False {
            }
            frame True {
              n254 = call "ASYNC_Adam_server.vi"("Values"=w610, "Channel Names"=w609) -> ("Scan Comments"=w607:string[])  [unwired: 1 in, 2 out]
              n255 = Index Array(array=w607, index=0) -> (element=w606:string)
            }
          }
        }
      }
      frame #18 {
        # "To automatically control the request for the University Stall chiller to run."
        n256 = while {
          tunnel: w615 -> [w623]
          tunnel: w614 -> [w624]
          shift-right: [w618] -> _
          shift-left: _ -> [w633]
          shift-left: _ -> [w632]
          shift-left: _ -> [w631]
          tunnel: [w617] -> w613
          tunnel: [w616] -> w612
          stop <- FALSE continue-if-true
          n257 = Build Array("EnFlo_Tunnel:Chiller_Pump:Enable" ("Desired Ch to Read"), "Aero_Tunnel:Cooling_Pump:Enable" ("Desired Ch to Read")) -> (w625:string[])
          n258 = call "Read_Earlier_Channels.vi"("Present scan array"=w623, "Ch names"=w624, "Desired Channels"=w625) -> ("Scan comments"=w616:string, "Index 0"=w622:dbl, "Index 1"=w621:dbl)  [unwired: 3 out]
          n259 = Build Array(w622, w621) -> (w620:dbl[])
          n260 = Greater?(x=w620, y=0.5) -> (0:w619:bool[])
          n261 = Or Array Elements(Boolean array=w619) -> (logical OR=w618:bool)
          n262 = Compound Arithmetic op=AND(w618, w633, invert w632, invert w631) -> (w629:bool)
          n263 = Compound Arithmetic op=AND(invert w618, invert w633, w632, w631) -> (w630:bool)
          n264 = Or(x=w629, y=w630) -> (x .or. y?=w628:bool)
          n265 = case shown="True" w628 {
            tunnel: w618 -> [_ w642]
            tunnel: [string[] [] ("Scan Comments") w637] -> w617
            frame False {
            }
            frame True {
              n266 = case shown="False" w642 {
                tunnel: [string[] ["University:Chilled Water:Requested"] ("Channel Names") string[] ["University:Chilled Water:Requested"] ("Channel Names")] -> w641
                tunnel: [1.0 ("y") 0.0 ("y")] -> w638
                frame True {
                }
                frame False {
                }
              }
              n267 = Array Size(array=w641) -> (size(s)=w639:i32)
              n268 = Initialize Array(w638, w639) -> (w640:dbl[])
              n269 = call "ASYNC_Adam_server.vi"("Values"=w640, "Channel Names"=w641) -> ("Scan Comments"=w637:string[])  [unwired: 1 in, 2 out]
            }
          }
        }
        n270 = Concatenate Strings(w613, w612) -> (w611:string)
      }
      frame #19 {
        # "Exercise the floor cooling valve once a week"
        n271 = while {
          shift-right: [w651] -> _
          shift-left: _ -> [w656]
          tunnel: w649 -> [w651]
          tunnel: w648 -> [w653]
          tunnel: [w650] -> w647
          stop <- TRUE stop-if-true
          n272 = Not Equal?(x=w651, y=w656) -> (x != y?=w654:bool)
          n273 = Compound Arithmetic op=AND(w654, w653) -> (w652:bool)
          n274 = case shown="True" w652 {
            tunnel: w651 -> [_ w663]
            tunnel: ["" w658] -> w650
            frame False {
            }
            frame True {
              n275 = Select(t=1.0, s=w663, f=0.0) -> (s? t:f=w664:dbl)
              n276 = Build Array(w664) -> (w667:dbl[])
              n277 = Build Array("EnFlo_Tunnel:Floor_Cooling:Enable") -> (w666:string[])
              n278 = call "ASYNC_Adam_server.vi"("Values"=w667, "Channel Names"=w666) -> ("Scan Comments"=w659:string[])  [unwired: 1 in, 2 out]
              n279 = Index Array(array=w659, index=0) -> (element=w658:string)
            }
          }
        }
      }
      frame #20 {
        n280 = Concatenate Strings(w673, w674, w675, w676, w677, w678, w679, w686, w685, w684, w683, w682, w681, w680, w671, w670, w669, w668) -> (→"Scan comment":string)
      }
    }
  }
